vi "MixtureControl.vi"(1 "%CO2":dbl, 2 "VISA resource name":refnum<visa-resource-name>="COM1") -> ()   [LabVIEW 2009]
uses:
  <vilib>/Instr/_visa.llb/VISA Configure Serial Port (Instr).vi
panel:
  out "CO2high":dbl
  out "CO2low":dbl
  out "H2":dbl
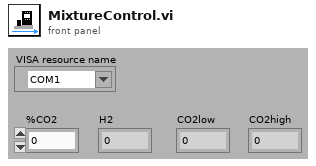
[diagram p1: front panel]
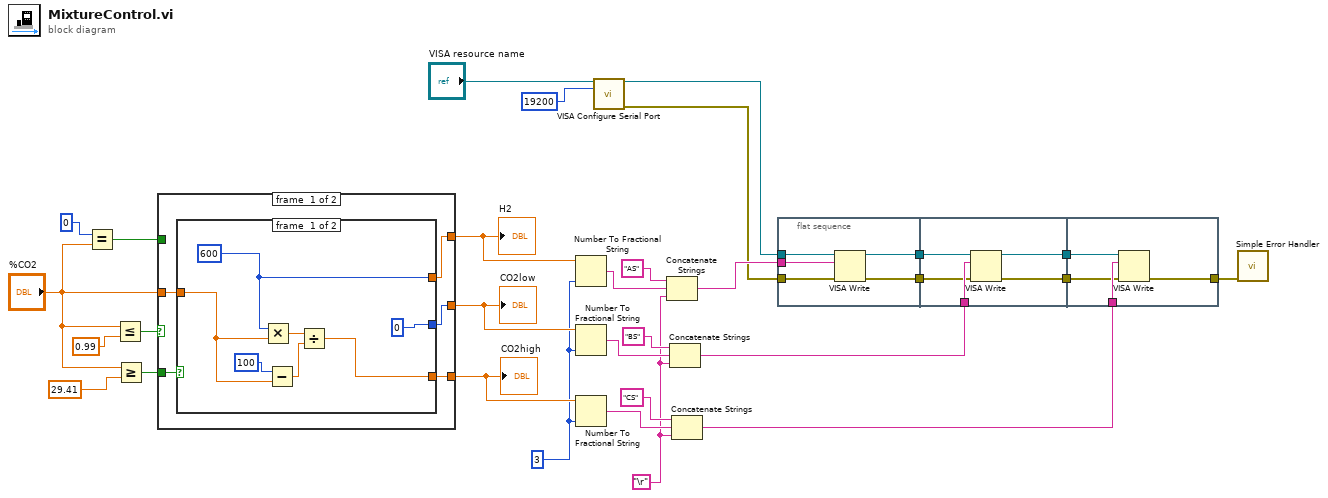
[diagram p0: block diagram]
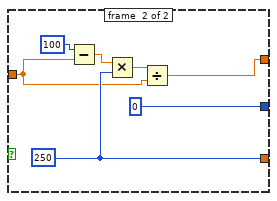
[diagram p2: hidden frame]
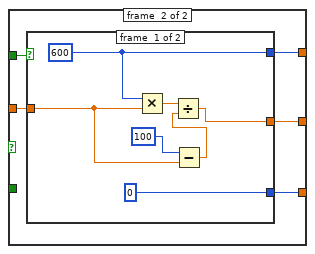
[diagram p3: hidden frame]
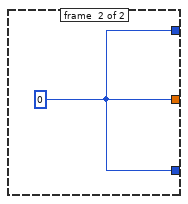
[diagram p4: hidden frame]
diagram:
  w1 = "\r"
  w11 = 3
  n1 = Equal?(x=0, y="%CO2") -> (x = y?=w7:bool)
  n2 = Less Or Equal?(x="%CO2", y=0.99) -> (x <= y?=w29:bool)
  n3 = Greater Or Equal?(x="%CO2", y=29.41) -> (x >= y?=w27:bool)
  n4 = case shown="False" w29 {
    tunnel: w27 -> [w35 _]
    tunnel: [w34 w53] -> w21
    tunnel: [w33 w54] -> w23
    tunnel: "%CO2" -> [w31 w51]
    tunnel: [w32 w52] -> w22
    tunnel: w7 -> [_ w50]
    frame #0 {
      n5 = case shown="True" w35 {
        tunnel: [w40 w43] -> w34
        tunnel: [w39 w46] -> w33
        tunnel: [0 0] -> w32
        tunnel: w31 -> [w36 w44]
        frame #0 {
          w40 = 600
          n6 = Multiply(x=w40, y=w36) -> (x*y=w41:dbl)
          n7 = Subtract(x=100, y=w36) -> (x-y=w37:dbl)
          n8 = Divide(x=w41, y=w37) -> (x/y=w39:dbl)
        }
        frame #1 {
          w46 = 250
          n9 = Subtract(x=100, y=w44) -> (x-y=w47:dbl)
          n10 = Multiply(x=w47, y=w46) -> (x*y=w45:dbl)
          n11 = Divide(x=w45, y=w44) -> (x/y=w43:dbl)
        }
      }
    }
    frame #1 {
      n12 = case shown="False" w50 {
        tunnel: [0 w62] -> w54
        tunnel: [w60 w62] -> w53
        tunnel: [w58 w62] -> w52
        tunnel: w51 -> [w56 _]
        frame #0 {
          w60 = 600
          n13 = Multiply(x=w60, y=w56) -> (x*y=w59:dbl)
          n14 = Subtract(x=100, y=w56) -> (x-y=w55:dbl)
          n15 = Divide(x=w59, y=w55) -> (x/y=w58:dbl)
        }
        frame #1 {
          w62 = 0
        }
      }
    }
  }
  "H2" <- w21
  "CO2low" <- w22
  "CO2high" <- w23
  n16 = Number To Fractional String(number=w21, precision (6)=w11) -> (F-format string=w20:string)  [unwired: 2 in]
  n17 = Number To Fractional String(number=w22, precision (6)=w11) -> (F-format string=w19:string)  [unwired: 2 in]
  n18 = Number To Fractional String(number=w23, precision (6)=w11) -> (F-format string=w18:string)  [unwired: 2 in]
  n19 = call-poly "VISA Configure Serial Port"("VISA resource name"="VISA resource name", "baud rate (9600)"=19200) -> ("VISA resource name out"=w3:refnum<visa-resource-name>, "error out"=w2:errorcluster)  [unwired: 4 in, 8 out]
  n20 = Concatenate Strings("AS", w20, w1) -> (w15:string)
  n21 = Concatenate Strings("BS", w19, w1) -> (w24:string)
  n22 = Concatenate Strings("CS", w18, w1) -> (w12:string)
  n23 = flat-sequence {
    tunnel: [w67] -> w26
    tunnel: [w66] -> w17
    tunnel: w3 -> [w65]
    tunnel: w15 -> [w64]
    tunnel: w2 -> [w63]
    tunnel: w26 -> [w72]
    tunnel: [w71] -> w25
    tunnel: w24 -> [w70]
    tunnel: w17 -> [w69]
    tunnel: [w68] -> w16
    tunnel: w25 -> [w76]
    tunnel: w12 -> [w75]
    tunnel: w16 -> [w74]
    tunnel: [w73] -> w10
    frame #0 {
      n24 = VISA Write(VISA resource name=w65, write buffer=w64, error in (no error)=w63) -> (VISA resource name out=w67:refnum<visa-resource-name>, error out=w66:errorcluster)  [unwired: 1 out]
    }
    frame #1 {
      n25 = VISA Write(VISA resource name=w72, write buffer=w70, error in (no error)=w69) -> (VISA resource name out=w71:refnum<visa-resource-name>, error out=w68:errorcluster)  [unwired: 1 out]
    }
    frame #2 {
      n26 = VISA Write(VISA resource name=w76, write buffer=w75, error in (no error)=w74) -> (error out=w73:errorcluster)  [unwired: 2 out]
    }
  }
  n27 = call <vilib>:"Simple Error Handler.vi"("error in (no error)"=w10) -> ()  [unwired: 4 in, 5 out]
